vi "Event-Driven State Machine - Handle Error Locally.vi"() -> ()   [LabVIEW 2020]
uses:
  support/States.ctl
  support/State Machine Data.ctl
  <vilib>/DAQmx/read.llb/DAQmx Read (Analog 2D DBL NChan NSamp).vi
  <vilib>/DAQmx/write.llb/DAQmx Write (Analog DBL 1Chan 1Samp).vi
  <vilib>/DAQmx/create/channels.llb/DAQmx Create Channel (AI-Voltage-Basic).vi
  <vilib>/DAQmx/configure/timing.llb/DAQmx Timing (Sample Clock).vi
  <vilib>/DAQmx/miscellaneous.llb/DAQmx Fill In Error Info.vi
  <vilib>/Utility/file.llb/Write Delimited Spreadsheet (DBL).vi
  <vilib>/DAQmx/create/channels.llb/DAQmx Create Channel (AO-Voltage-Basic).vi
panel:
  in  "AO Voltage Channel":tag="PCI-6221/ao1"
  in  "Generate Stimulus":bool
  out "Threshold exceeded?":bool
  in  "Acquire":bool
  in  "Samples per channel":i32=100
  in  "Sample Rate (Hz)":dbl=1000.0
  in  "AI Voltage Channel":tag="PCI-6221/ai0, PCI-6221/ai2:3"
  in  "Threshold (rms)":dbl=1.0 min=0.0
  in  "Clear":bool
  in  "Exit":bool
  out "Graph":dbl[][](graph)
  # "Analysis"
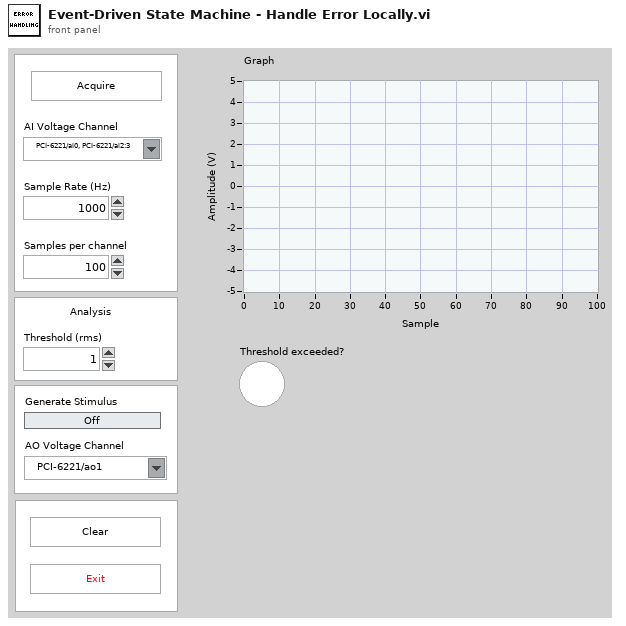
[diagram p1: front panel]
types:
  T1 = typedef "State Machine Data.ctl" = cluster{"Acquisition Data":dbl[][], "Stimulus Value":bool}
  T2 = typedef "States.ctl" = enum16{"Initialize", "Wait for Event", "Acquire", "Analyze", "Log", "Clear", "Update Graph", "Update Stumulus", "Exit"}
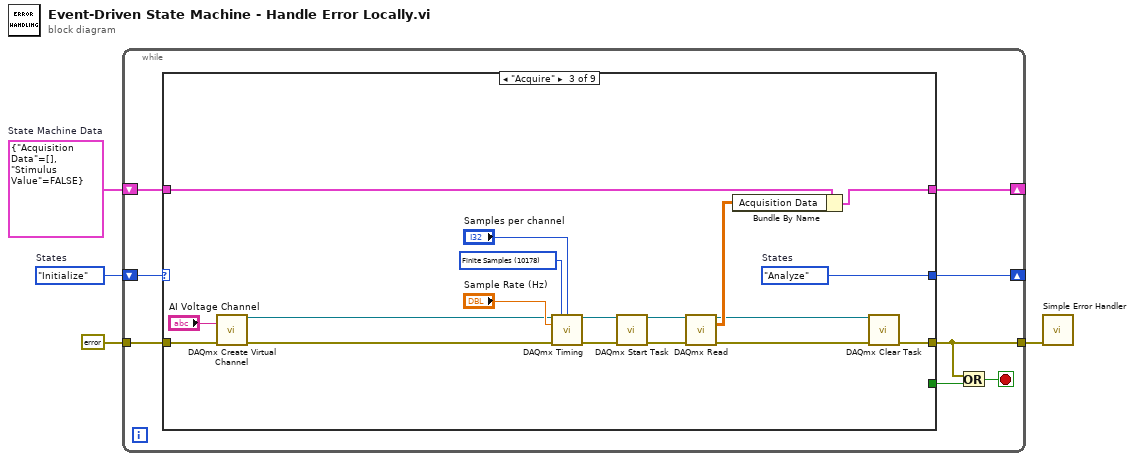
[diagram p0: block diagram]
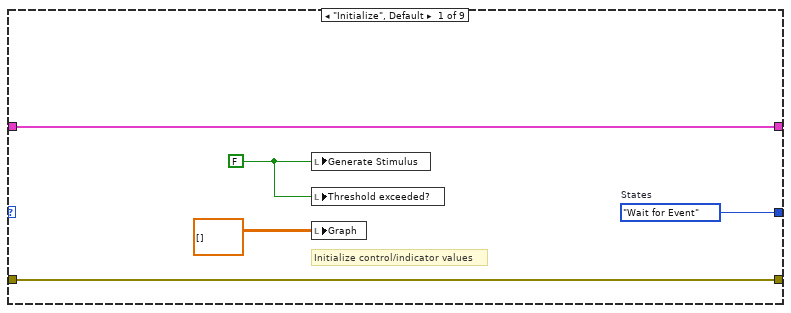
[diagram p2: hidden frame]
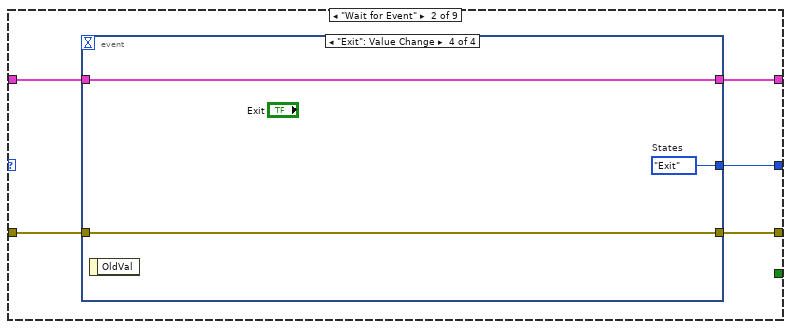
[diagram p3: hidden frame]
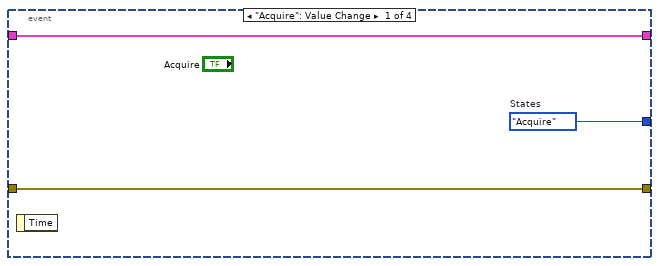
[diagram p4: hidden frame]
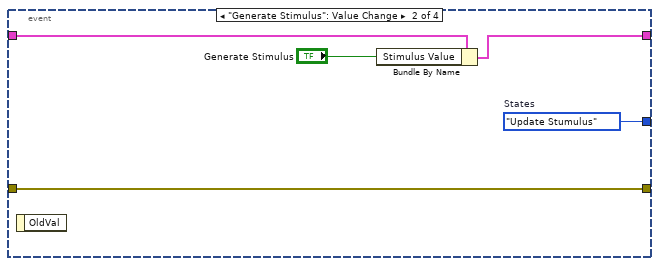
[diagram p5: hidden frame]
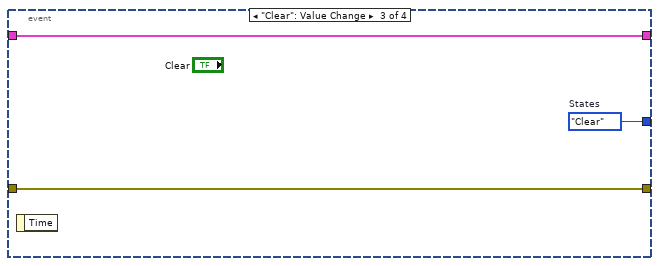
[diagram p6: hidden frame]
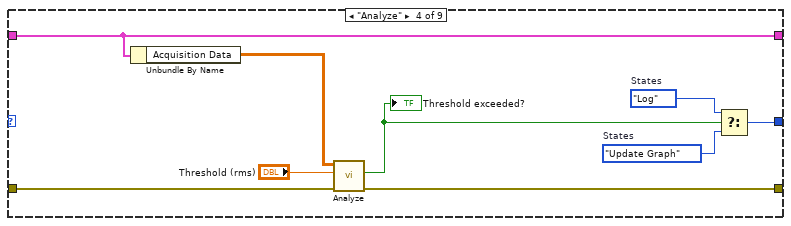
[diagram p7: hidden frame]
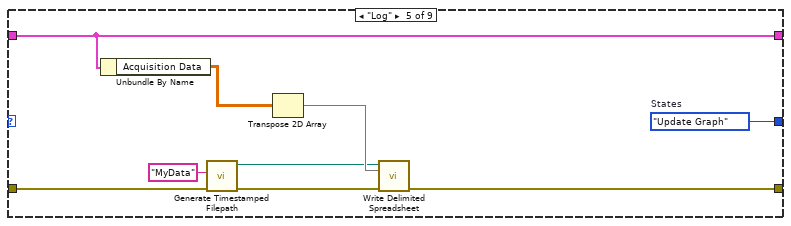
[diagram p8: hidden frame]
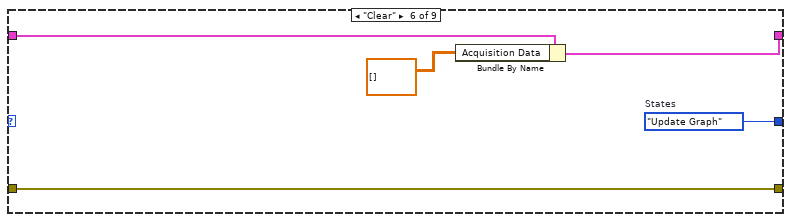
[diagram p9: hidden frame]
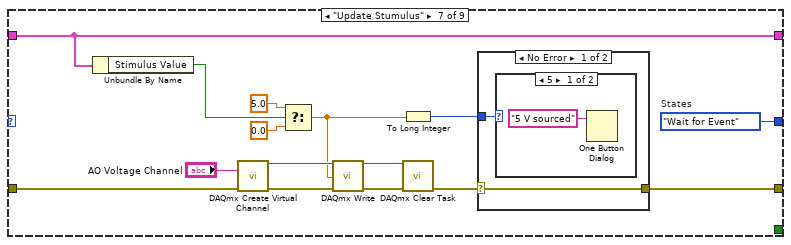
[diagram p10: hidden frame]
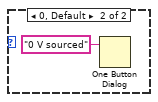
[diagram p11: hidden frame]
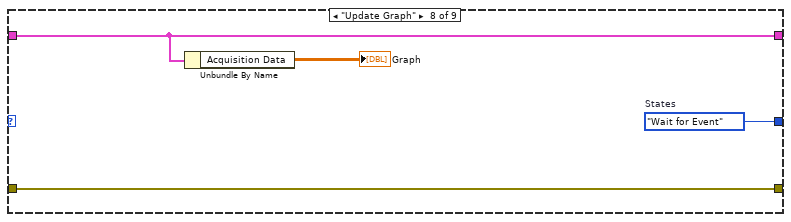
[diagram p13: hidden frame]
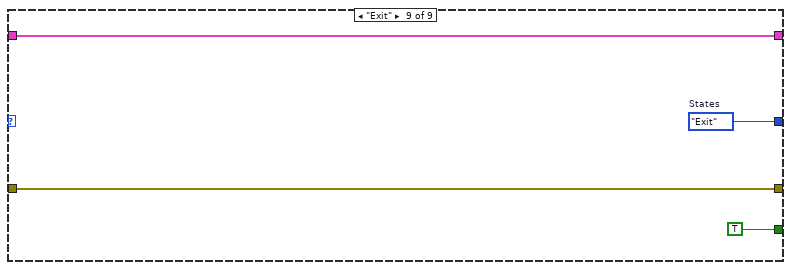
[diagram p14: hidden frame]
diagram:
  w4 = T1 {"Acquisition Data"=[], "Stimulus Value"=FALSE}  # State Machine Data
  w3 = States."Initialize"  # States
  n1 = while {
    tunnel: errorcluster {"status"=FALSE, "code"=0, "source"=""} ("error constant") -> [w11]
    tunnel: [w7] -> w1
    shift-right: [w9] -> _
    shift-left: w4 -> [w10]
    shift-right: [w8] -> _
    shift-left: w3 -> [w12]
    stop <- w6 stop-if-true
    n2 = case shown="\"Acquire\"" w12 {
      tunnel: w11 -> [w17 w20 w54 w62 w71 w77 w80 w100 w104]
      tunnel: [w17 w19 w49 w61 w65 w77 w78 w100 w104] -> w7
      tunnel: [w16 w21 w46 w63 w72 w75 w92 w101 w105] -> w9
      tunnel: w10 -> [w16 w22 w47 w63 w72 w76 w92 w101 w105]
      tunnel: [w15 w18 w48 w57 w64 w73 w81 w99 w102] -> w8
      tunnel: [_ _ _ _ _ _ _ _ TRUE] -> w5
      frame "Initialize", Default {
        w14 = FALSE
        w15 = States."Wait for Event"  # States
        # "Initialize control/indicator values"
        n3 = local write "Generate Stimulus"(w14) -> ()
        n4 = local write "Threshold exceeded?"(w14) -> ()
        n5 = local write "Graph"(dbl[][] []) -> ()
      }
      frame "Wait for Event" {
        n6 = event shown="[3] \"Exit\": Value Change" {
          selector: _ -> [_ _ _ _]
          dyn-events: _ -> [_ _ _ _]
          timeout: _ -> [_ _ _ _]
          tunnel: w22 -> [w25 w30 w33 w35]
          tunnel: [w25 w29 w33 w35] -> w21
          tunnel: w20 -> [w24 w26 w32 w36]
          tunnel: [w24 w26 w32 w36] -> w19
          tunnel: [w23 w27 w31 w34] -> w18
          event "Acquire": Value Change {
            w23 = States."Acquire"  # States
            n7 = event-data() -> ()  [unwired: 1 in, 1 out]
          }
          event "Generate Stimulus": Value Change {
            w27 = States."Update Stumulus"  # States
            n8 = event-data() -> ()  [unwired: 1 in, 1 out]
            n9 = Bundle By Name(cluster=w30, "Stimulus Value"="Generate Stimulus") -> (w29:T1)
          }
          event "Clear": Value Change {
            w31 = States."Clear"  # States
            n10 = event-data() -> ()  [unwired: 1 in, 1 out]
          }
          event "Exit": Value Change {
            w34 = States."Exit"  # States
            n11 = event-data() -> ()  [unwired: 1 in, 1 out]
          }
        }
      }
      frame "Acquire" {
        w45 = 10178 items=["Finite Samples"=10178, "Continuous Samples"=10123, "Hardware Timed Single Point"=12522] ("sample mode")
        w48 = States."Analyze"  # States
        n12 = call-poly <vilib>:"DAQmx Create Virtual Channel.vi"("physical channels"="AI Voltage Channel", "error in"=w54) -> ("task out"=w40:refnum<k21>, "error out"=w53:errorcluster)  [unwired: 12 in]
        n13 = call-poly <vilib>:"DAQmx Timing.vi"("task/channels in"=w40, "sample mode"=w45, "samples per channel"="Samples per channel", "rate"="Sample Rate (Hz)", "error in"=w53) -> ("task out"=w39:refnum<k21>, "error out"=w52:errorcluster)  [unwired: 9 in]
        n14 = call <vilib>:"DAQmx Start Task.vi"("task/channels in"=w39, "error in"=w52) -> ("task out"=w38:refnum<k21>, "error out"=w51:errorcluster)  [unwired: 12 in]
        n15 = call-poly <vilib>:"DAQmx Read.vi"("task/channels in"=w38, "error in"=w51) -> ("task out"=w37:refnum<k21>, "data"=w41:dbl[][], "error out"=w50:errorcluster)  [unwired: 11 in]
        n16 = Bundle By Name(cluster=w47, "Acquisition Data"=w41) -> (w46:T1)
        n17 = call <vilib>:"DAQmx Clear Task.vi"("task in"=w37, "error in"=w50) -> ("error out"=w49:errorcluster)  [unwired: 13 in]
      }
      frame "Analyze" {
        w58 = States."Update Graph"  # States
        w59 = States."Log"  # States
        n18 = Unbundle By Name(w63) -> ("Acquisition Data"=w60:dbl[][])
        n19 = call "Analyze.vi"("Error In"=w62, "Treshold (rms)"="Threshold (rms)", "N-Channel Data (2D DBL)"=w60) -> ("Error Out"=w61:errorcluster, "Threshold exceeded?"=w55:bool)  [unwired: 5 in, 2 out]
        "Threshold exceeded?" <- w55
        n20 = Select(t=w59, s=w55, f=w58) -> (s? t:f=w57:T2)
      }
      frame "Log" {
        w64 = States."Update Graph"  # States
        n21 = Unbundle By Name(w72) -> ("Acquisition Data"=w69:dbl[][])
        n22 = call "Generate Timestamped Filepath.vi"("Error In"=w71, "appended filename"="MyData") -> ("Error Out"=w66:errorcluster, "timestamped relative filepath"=w67:path)  [unwired: 8 in]
        n23 = Transpose 2D Array(2D array=w69) -> (transposed array=w68:dbl[][])
        n24 = call-poly <vilib>:"Write Delimited Spreadsheet.vi"("file path (dialog if empty)"=w67, "2D data"=w68, "error in (no error)"=w66) -> ("error out"=w65:errorcluster)  [unwired: 11 in, 1 out]
      }
      frame "Clear" {
        w73 = States."Update Graph"  # States
        n25 = Bundle By Name(cluster=w76, "Acquisition Data"=dbl[][] []) -> (w75:T1)
      }
      frame "Update Stumulus" {
        w81 = States."Wait for Event"  # States
        n26 = Unbundle By Name(w92) -> ("Stimulus Value"=w82:bool)
        n27 = call-poly <vilib>:"DAQmx Create Virtual Channel.vi"("physical channels"="AO Voltage Channel", "error in"=w80) -> ("task out"=w89:refnum<k21>, "error out"=w88:errorcluster)  [unwired: 12 in]
        n28 = Select(t=5.0, s=w82, f=0.0) -> (s? t:f=w84:dbl)
        n29 = call-poly <vilib>:"DAQmx Write.vi"("task/channels in"=w89, "data"=w84, "error in"=w88) -> ("task out"=w87:refnum<k21>, "error out"=w86:errorcluster)  [unwired: 10 in, 1 out]
        n30 = To Long Integer(number=w84) -> (32bit integer=w83:i32)
        n31 = call <vilib>:"DAQmx Clear Task.vi"("task in"=w87, "error in"=w86) -> ("error out"=w79:errorcluster)  [unwired: 13 in]
        n32 = case shown="No Error" w79 {
          selector: w79 -> [w93 w97]
          tunnel: w83 -> [w94 _]
          tunnel: [w93 w97] -> w78
          frame No Error {
            n33 = case shown="5" w94 {
              frame 5 {
                n34 = One Button Dialog(message="5 V sourced") -> ()  [unwired: 1 in, 1 out]
              }
              frame 0, Default {
                n35 = One Button Dialog(message="0 V sourced") -> ()  [unwired: 1 in, 1 out]
              }
            }
          }
          frame Error {
          }
        }
      }
      frame "Update Graph" {
        w99 = States."Wait for Event"  # States
        n36 = Unbundle By Name(w101) -> ("Acquisition Data"=→"Graph":dbl[][])
      }
      frame "Exit" {
        w102 = States."Exit"  # States
      }
    }
    n37 = Or(x=w7, y=w5) -> (x .or. y?=w6:bool)
  }
  n38 = call <vilib>:"Simple Error Handler.vi"("error in (no error)"=w1) -> ()  [unwired: 4 in, 5 out]
